vi "Transform.vi"(8 "error in (no error)":errorcluster, 11 "XRay Beam in":refnum<class "XRay Beam.lvclass">) -> (0 "error out":errorcluster, 3 "XRay Beam out":refnum<class "XRay Beam.lvclass">)   [LabVIEW 2026, in "XRay Beam.lvclass"]
uses:
  XRay Beam.lvclass
  XRay Beam.lvclass/XRay Beam.ctl
  XRay CArm/XRay CArm.lvclass/XRay CArm.ctl
  <vilib>/picture/3D Picture Control/NI_3D Picture Control.lvlib
  XRay CArm/XRay CArm.lvclass
panel:
  out "error out 2":errorcluster
  out "C Arm Height":sgl
  out "C Arm Angle":dbl
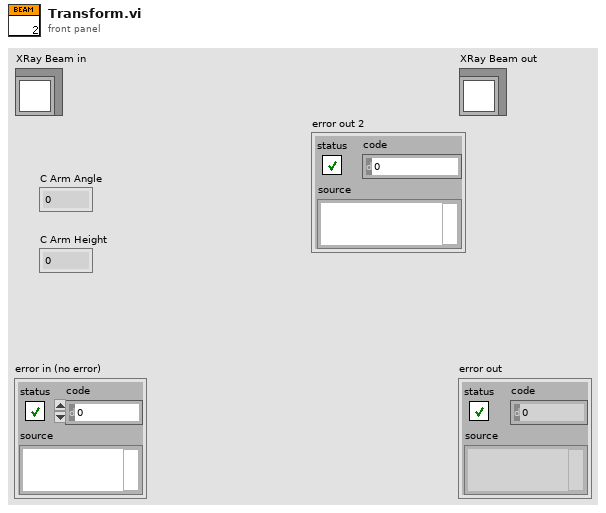
[diagram p1: front panel]
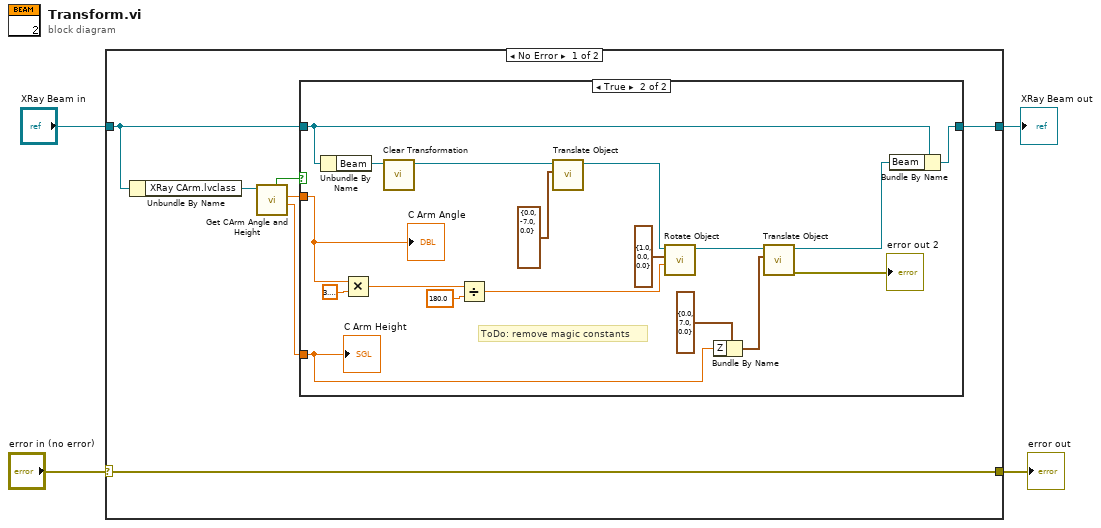
[diagram p0: block diagram]
diagram:
  n1 = case shown="No Error" "error in (no error)" {
    selector: "error in (no error)" -> [w11 w32]
    tunnel: [w11 w32] -> w3
    tunnel: [w10 w31] -> w1
    tunnel: "XRay Beam in" -> [w9 w31]
    frame No Error {
      n2 = Unbundle By Name(w9) -> ("XRay CArm.lvclass"=w8:refnum<class "XRay CArm.lvclass">)
      n3 = call "Get CArm Angle and Height.vi"("XRay CArm in"=w8) -> ("CArm Height"=w6:sgl, "CArm Angle"=w7:sgl, "Pos Changed"=w5:bool)  [unwired: 6 in, 2 out]
      n4 = case shown="True" w5 {
        tunnel: [w12 w30] -> w10
        tunnel: w9 -> [w12 w29]
        tunnel: w7 -> [_ w28]
        tunnel: w6 -> [_ w27]
        frame False {
        }
        frame True {
          # "ToDo: remove magic constants"
          n5 = Unbundle By Name(w29) -> ("Beam"=w23:refnum<vi>)
          n6 = Multiply(x=w28, y=3.141592653589793) -> (x*y=w25:dbl)
          n7 = call <vilib>:"Clear Transformation.vi"("Object Refnum In"=w23) -> ("Object Refnum Out"=w18:refnum<vi>)  [unwired: 1 in, 9 out]
          n8 = Divide(x=w25, y=180.0) -> (x/y=w22:dbl)
          n9 = call <vilib>:"Translate Object.vi"("Translation"=cluster{"X":sgl, "Y":sgl, "Z":sgl} {"X"=0.0, "Y"=-7.0, "Z"=0.0} ("Translation 3"), "Scene.Object In"=w18) -> ("Scene.Object Out"=w17:refnum<vi>)  [unwired: 8 in, 1 out]
          n10 = call <vilib>:"Rotate Object.vi"("Angle"=w22, "Axis"=cluster{"X":sgl, "Y":sgl, "Z":sgl} {"X"=1.0, "Y"=0.0, "Z"=0.0}, "Scene.Object In"=w17) -> ("Scene.Object Out"=w21:refnum<vi>)  [unwired: 7 in, 1 out]
          n11 = Bundle By Name(cluster=cluster{"X":sgl, "Y":sgl, "Z":sgl} {"X"=0.0, "Y"=7.0, "Z"=0.0} ("Translation 2"), "Z"=w27) -> (w15:cluster{"X":sgl, "Y":sgl, "Z":sgl})
          n12 = call <vilib>:"Translate Object.vi"("Translation"=w15, "Scene.Object In"=w21) -> ("error out"=→"error out 2":errorcluster, "Scene.Object Out"=w20:refnum<vi>)  [unwired: 8 in]
          n13 = Bundle By Name(cluster=w29, "Beam"=w20) -> (w30:refnum<class "XRay Beam.lvclass">)
          "C Arm Angle" <- w28
          "C Arm Height" <- w27
        }
      }
    }
    frame Error {
    }
  }
  "error out" <- w3
  "XRay Beam out" <- w1
